vi "Excel Get Data (dbl).vi"(0 "report in":refnum<class "NI_report.lvclass">, 5 "data type":dbl format="%.2f", 7 "start (0, 0)":cluster{"start row":i32, "start column":i32}, 11 "error in (no error)":errorcluster, 12 "name (\"\")":string) -> (4 "report out":refnum<class "NI_report.lvclass">, 8 "data":dbl format="%.2f", 15 "error out":errorcluster)   [LabVIEW 2016, in "NI_Excel.lvclass"]
doc: "Retrieves data from the current worksheet. The data type you wire to the <B>data type</B> input determines the polymorphic instance to use."
uses:
  <vilib>/Utility/NIReport.llb/Excel/NI_Excel.lvclass
  <vilib>/Utility/NIReport.llb/NI_report.lvclass
  C:/Program Files (x86)/National Instruments/LabVIEW 2016/vi.lib/Utility/NIReport.llb/NI_report.lvclass
  <vilib>/Utility/NIReport.llb/Excel/NI_Excel.lvclass/NI_Excel.ctl
  <vilib>/Utility/NIReport.llb/NI_ReportGenerationCore.lvlib
  <vilib>/addons/_office/NI_ReportGenerationToolkit.lvlib
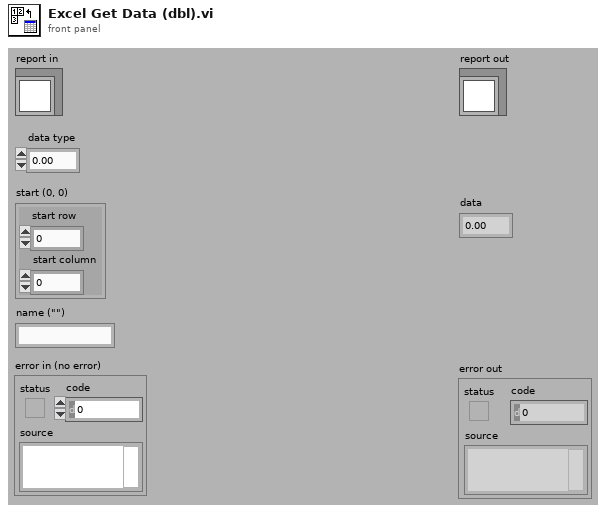
[diagram p1: front panel]
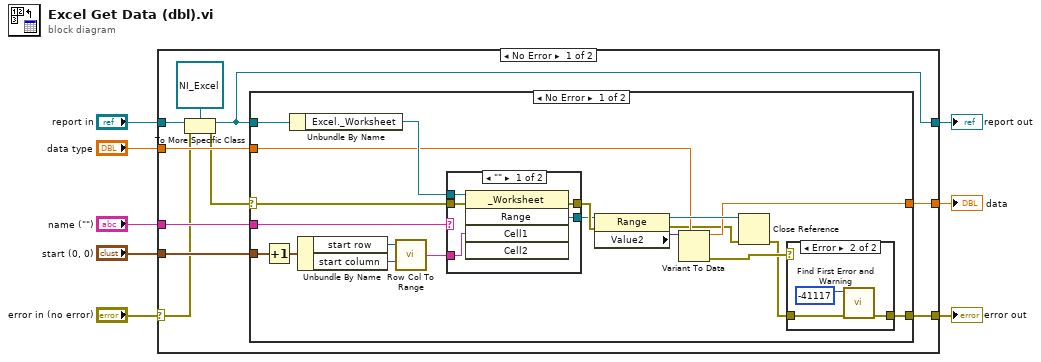
[diagram p0: block diagram]
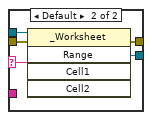
[diagram p3: hidden frame]
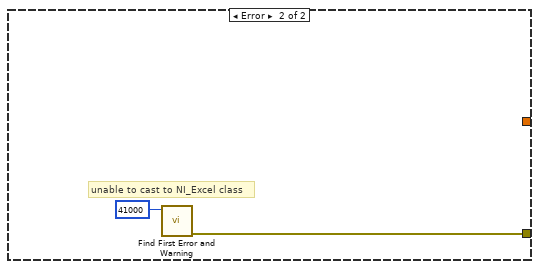
[diagram p4: hidden frame]
diagram:
  n1 = case shown="No Error" "error in (no error)" {
    selector: "error in (no error)" -> [w9 w55]
    tunnel: [w14 w55] -> w7
    tunnel: [w11 w54] -> w5
    tunnel: "report in" -> [w12 w54]
    tunnel: "name (\"\")" -> [w18 _]
    tunnel: "start (0, 0)" -> [w17 _]
    tunnel: "data type" -> [w16 _]
    tunnel: [w15 _] -> w1
    frame No Error {
      n2 = To More Specific Class(target class=refnum<class "NI_Excel.lvclass"> refnum ("report in"), reference=w12, error in=w9) -> (specific class reference=w11:refnum<class "NI_Excel.lvclass">, error out=w10:errorcluster)
      n3 = case shown="No Error" w10 {
        selector: w10 -> [w23 _]
        tunnel: w18 -> [w28 _]
        tunnel: w17 -> [w27 _]
        tunnel: w16 -> [w26 _]
        tunnel: [w25 _] -> w15
        tunnel: [w19 w52] -> w14
        tunnel: w11 -> [w24 _]
        frame No Error {
          n4 = Increment(x=w27) -> (x+1=w36:cluster{"start row":i32, "start column":i32})
          n5 = Unbundle By Name(w24) -> ("Excel._Worksheet"=w29:refnum<k7>)
          n6 = Unbundle By Name(w36) -> ("start row"=w35:i32, "start column"=w34:i32)
          n7 = call <vilib>:"Row Col To Range.vi"("Column"=w34, "Row"=w35) -> ("Output String"=w37:string)
          n8 = case shown="\"\"" w28 {
            selector: w28 -> [_ w47]
            tunnel: w29 -> [w46 w51]
            tunnel: [w45 w50] -> w30
            tunnel: w37 -> [w42 _]
            tunnel: w23 -> [w44 w49]
            tunnel: [w43 w48] -> w32
            frame "" {
              n9 = invoke class="_Worksheet" method="Range"(reference=w46, error in=w44, "Cell1"=w42) -> (error out=w43:errorcluster, "Range"=w45:refnum<k7>)  [unwired: 2 in, 3 out]
            }
            frame Default {
              n10 = invoke class="_Worksheet" method="Range"(reference=w51, error in=w49, "Cell1"=w47) -> (error out=w48:errorcluster, "Range"=w50:refnum<k7>)  [unwired: 2 in, 3 out]
            }
          }
          n11 = property class="Range"(reference=w30, error in=w32) -> (reference out=w33:refnum<k7>, error out=w22:errorcluster, "Value2"=w31:variant)
          n12 = Variant To Data(type=w26, Variant=w31) -> (data=w25:dbl, error out=w21:errorcluster)  [unwired: 1 in]
          n13 = Close Reference(reference=w33, error in (no error)=w22) -> (error out=w20:errorcluster)
          n14 = case shown="Error" w21 {
            tunnel: [w38 w40] -> w19
            tunnel: w20 -> [w38 w39]
            frame No Error {
            }
            frame Error {
              n15 = call <vilib>:"Find First Error and Warning.vi"("error in (no error)"=w39, "error code"=-41117) -> ("error out"=w40:errorcluster)  [unwired: 1 in, 4 out]
            }
          }
        }
        frame Error {
          # "unable to cast to NI_Excel class"
          n16 = call <vilib>:"Find First Error and Warning.vi"("error code"=41000) -> ("error out"=w52:errorcluster)  [unwired: 2 in, 4 out]
        }
      }
    }
    frame Error {
    }
  }
  "error out" <- w7
  "report out" <- w5
  "data" <- w1
